vi "Login 2.0.vi"() -> (0 "quit led":bool, 1 "UTENTE":string, 2 "?":bool)   [LabVIEW 2012]
uses:
  <vilib>/Utility/file.llb/Read From Spreadsheet File (string).vi
panel:
  in  "?":bool
  out "?":string
  in  "?":bool
  in  "Username":string
  in  "Password":string
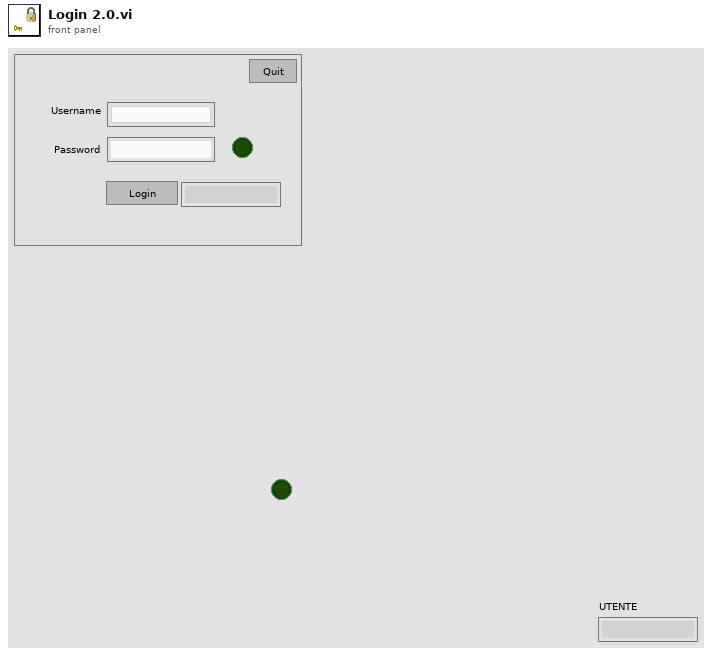
[diagram p1: front panel]
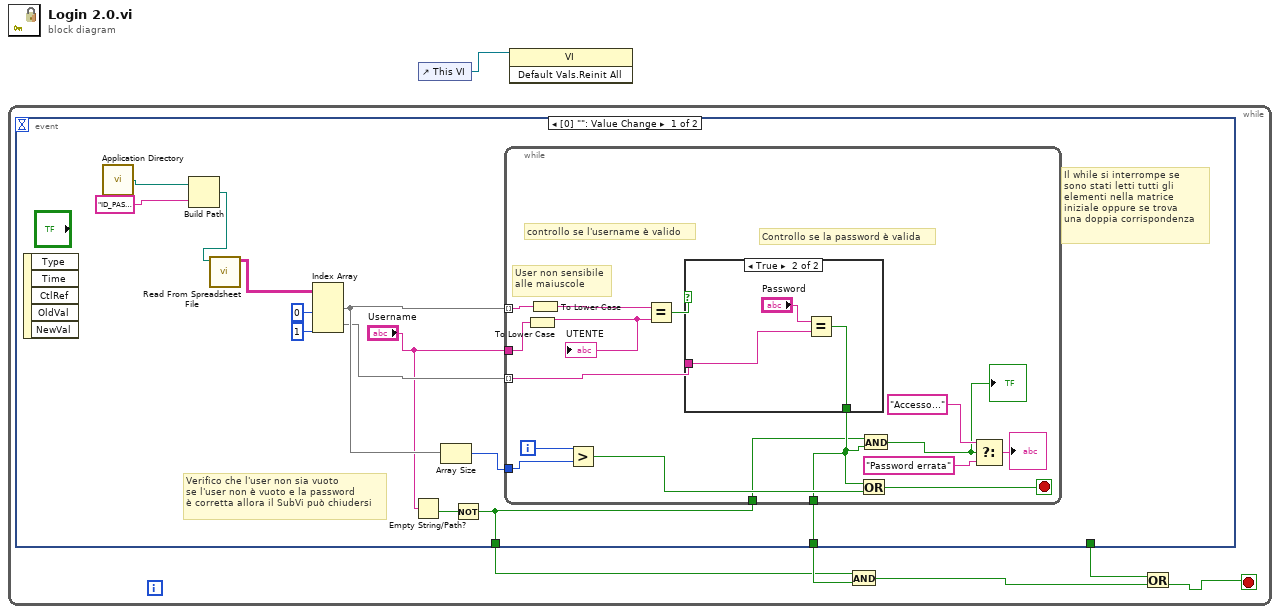
[diagram p0: block diagram]
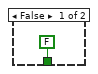
[diagram p2: hidden frame]
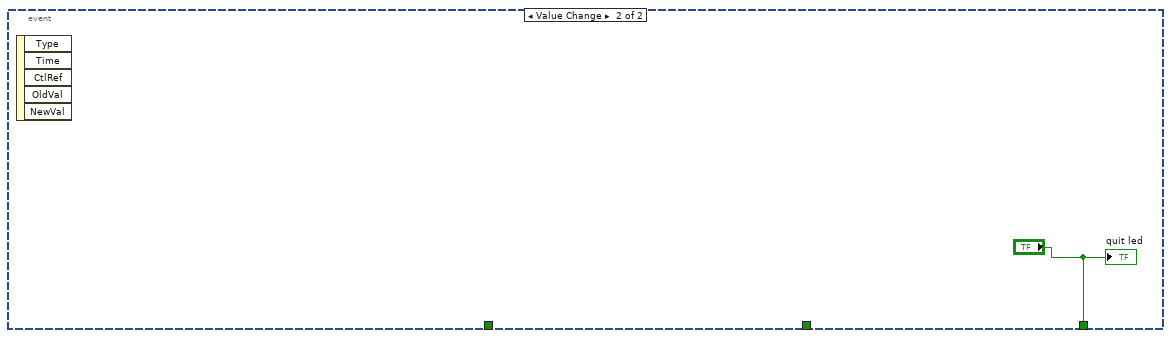
[diagram p3: hidden frame]
diagram:
  n1 = while {
    stop <- w3 stop-if-true
    n2 = event shown="[0] \"\": Value Change" {
      selector: _ -> [_ _]
      dyn-events: _ -> [_ _]
      timeout: _ -> [_ _]
      tunnel: [w13 _] -> w6
      tunnel: [w10 _] -> w5
      tunnel: [_ "?"] -> w2
      event Value Change {
        # "Verifico che l'user non sia vuoto\nse l'user non è vuoto e la password\nè corretta allora il SubVi può chiudersi"
        # "Il while si interrompe se\nsono stati letti tutti gli \nelementi nella matrice \niniziale oppure se trova\nuna doppia corrispondenza"
        n3 = event-data() -> ()  [unwired: 1 in, 5 out]
        n4 = call <vilib>:"Application Directory.vi"() -> ("Application Directory"=w9:path)
        n5 = Build Path(base path=w9, name or relative path="ID_PASS.txt") -> (appended path=w7:path)
        n6 = call-poly <vilib>:"Read From Spreadsheet File.vi"("file path (dialog if empty)"=w7) -> ("all rows"=w17:string[][])  [unwired: 6 in, 4 out]
        n7 = Index Array(array=w17, index (col) #1=0 ("disabled index (col)"), index (col) #2=1 ("index (col)")) -> (element #1=w16:string[], element #2=w15:string[])  [unwired: 2 in]
        n8 = Empty String/Path?(string/path="Username") -> (empty?=w11:bool)
        n9 = Array Size(array=w16) -> (size(s)=w14:i32)
        n10 = Not(x=w11) -> (.not. x?=w10:bool)
        n11 = while {
          tunnel: "Username" -> [w34]
          tunnel: w16 -> [w35] mode=indexing
          tunnel: w15 -> [w33] mode=indexing
          tunnel: w14 -> [w27]
          tunnel: [w22] -> w13
          tunnel: w10 -> [w21]
          i -> [w26]
          stop <- w24 stop-if-true
          # "Controllo se la password è valida"
          # "controllo se l'username è valido"
          # "User non sensibile\nalle maiuscole"
          n12 = To Lower Case(string=w34) -> (all lower case string=w23:string)
          "UTENTE" <- w23
          n13 = To Lower Case(string=w35) -> (all lower case string=w28:string)
          n14 = Greater?(x=w26, y=w27) -> (0:w25:bool)
          n15 = Equal?(x=w28, y=w23) -> (x = y?=w32:bool)
          n16 = case shown="True" w32 {
            tunnel: w33 -> [_ w38]
            tunnel: [FALSE w37] -> w22
            frame False {
            }
            frame True {
              n17 = Equal?(x="Password", y=w38) -> (x = y?=w37:bool)
            }
          }
          n18 = Or(x=w22, y=w25) -> (x .or. y?=w24:bool)
          n19 = And(x=w21, y=w22) -> (x .and. y?=w20:bool)
          "?" <- w20
          n20 = Select(t="Accesso...", s=w20, f="Password errata") -> (s? t:f=→"?":string)
        }
      }
      event Value Change {
        n21 = event-data() -> ()  [unwired: 1 in, 5 out]
        "quit led" <- "?"
      }
    }
    n22 = And(x=w5, y=w6) -> (x .and. y?=w4:bool)
    n23 = Or(x=w2, y=w4) -> (x .or. y?=w3:bool)
  }
  n24 = control-ref of="This VI"() -> (w1:refnum<vi>)
  n25 = invoke class="VI" method="Default Vals.Reinit All"(reference=w1) -> ()  [unwired: 2 in, 3 out]
